vi "Run Bfr Tx - Check Valid Buffer.vi"(8 "error in (no error)":errorcluster, 11 "Tx Loop Data in":T1={"General Resources"={"Packet Name"="", "Packet ID"=0, "Local IP Address"="", "Local Port"=0, "Multicast"=FALSE, "Multicast IP Address"=0, "Header Info"=[], "Byte Order"=enum."big-endian, network order", "Channel Data Types"=[], "Duplex Packets"=refnum}, "Header Details"={"Packet Size"=0, "Protocol Revision"=0, "System Definition Version"=0, "Source Node Name"="", "Packet ID"=0, "Number of Channels"=0, "Static Header Size"=0, "Total Header Size"=0}, "Buffer Resources"={"Data Buffer"=0, "Pointer Encoding"=enum."Direct Encoding", "Buffer Size"=0, "Raw Buffer Data"=[], "Is Buffered"=FALSE, "External Buffer"=FALSE, "Prepend Header"=FALSE, "Valid Buffer"=FALSE}, "Runtime Resources"={"Connection ID"=refnum, "Transmit Option"=enum."Always", "Destination IP Address"=0, "Destination Port"=0, "Multicast IP Address"=0, "TTL"=0, "Multicast"=FALSE, "Port as Channel"=FALSE, "ExecutionConfig"={"Loop Period"=0, "RT Loop Period"=-2, "Untimed Period"=0, "Target Processor"=0, "Priority"=0, "Thread Management"=enum."Untimed (Default)"}}, "Echo Resources"={"Transmit Echo Option"=enum."PCL Reset", "Packet Count"=0.0, "Counter Increment"=0.0, "Transmit Values"=[]}, "Buffer Option Support"={"Buffer Option"=enum."Static Buffer", "Sim Option"=enum."No Simulation"}, "Channel Resources"={"Transmit Flag"=refnum, "Transmit Echo"=refnum, "Transmit Bytes"=refnum, "Port Channel"=refnum, "Buffer (External)"=refnum, "Buffer (Local)"=refnum, "Timestamp"=refnum}, "Debug Resources"={"Debug Mode"=FALSE, "Debug Log File"=refnum, "Packet Name"=""}} {"Buffer Resources"."Data Buffer" format="%016x"}) -> (0 "error out":errorcluster, 3 "Tx Loop Data out":T1={"General Resources"={"Packet Name"="", "Packet ID"=0, "Local IP Address"="", "Local Port"=0, "Multicast"=FALSE, "Multicast IP Address"=0, "Header Info"=[], "Byte Order"=enum."big-endian, network order", "Channel Data Types"=[], "Duplex Packets"=refnum}, "Header Details"={"Packet Size"=0, "Protocol Revision"=0, "System Definition Version"=0, "Source Node Name"="", "Packet ID"=0, "Number of Channels"=0, "Static Header Size"=0, "Total Header Size"=0}, "Buffer Resources"={"Data Buffer"=0, "Pointer Encoding"=enum."Direct Encoding", "Buffer Size"=0, "Raw Buffer Data"=[], "Is Buffered"=FALSE, "External Buffer"=FALSE, "Prepend Header"=FALSE, "Valid Buffer"=FALSE}, "Runtime Resources"={"Connection ID"=refnum, "Transmit Option"=enum."Always", "Destination IP Address"=0, "Destination Port"=0, "Multicast IP Address"=0, "TTL"=0, "Multicast"=FALSE, "Port as Channel"=FALSE, "ExecutionConfig"={"Loop Period"=0, "RT Loop Period"=-2, "Untimed Period"=0, "Target Processor"=0, "Priority"=0, "Thread Management"=enum."Untimed (Default)"}}, "Echo Resources"={"Transmit Echo Option"=enum."PCL Reset", "Packet Count"=0.0, "Counter Increment"=0.0, "Transmit Values"=[]}, "Buffer Option Support"={"Buffer Option"=enum."Static Buffer", "Sim Option"=enum."No Simulation"}, "Channel Resources"={"Transmit Flag"=refnum, "Transmit Echo"=refnum, "Transmit Bytes"=refnum, "Port Channel"=refnum, "Buffer (External)"=refnum, "Buffer (Local)"=refnum, "Timestamp"=refnum}, "Debug Resources"={"Debug Mode"=FALSE, "Debug Log File"=refnum, "Packet Name"=""}} {"Buffer Resources"."Data Buffer" format="%016x"})   [LabVIEW 2016, in "UDP-Custom-Device Engine.lvlib"]
uses:
  UDP-Custom-Device Engine.lvlib
  Types/Engine - Buffered Tx Loop Data.ctl
  Types/Engine - General Resources.ctl
  <vilib>/NI Veristand/VeriStand Data/Typedefs/Typedefs.Data Types.ctl
  Shared/Types/Shared - Duplex Settings.ctl
  Shared/Types/Shared - Header Details.ctl
  Types/Engine - Buffer Resources.ctl
  Shared/Types/Shared - Pointer Encoding.ctl
  Types/Engine - Tx Runtime Resources.ctl
  Shared/Types/Shared - Transmit Flag Options.ctl
  Types/Engine - Execution Config.ctl
  Shared/Types/Shared - Thread Management.ctl
  Types/Engine - Tx Echo Resources.ctl
  Shared/Types/Shared - Transmit Echo Options.ctl
  Types/Engine - Buffered Tx Buffer Option Support.ctl
  Shared/Types/Shared - Transmit Buffer Options.ctl
  Shared/Types/Shared - Transmit Sim Options.ctl
  Types/Engine - Buffered Tx Channel Refs.ctl
  <vilib>/NI/NIVS Inline Async API/_Data Access Engine/Data Access Engine/Types/Read.DVR.ctl
  <vilib>/NI/NIVS Inline Async API/_Data Access Engine/Access Type Classes/Read/Read.lvclass
  <vilib>/NI/NIVS Inline Async API/_Data Access Engine/Data Access Engine/Types/Write.DVR.ctl
  <vilib>/NI/NIVS Inline Async API/_Data Access Engine/Access Type Classes/Write/Write.lvclass
  Types/Engine - Debug Resources.ctl
  <vilib>/NI/NIVS Inline Async API/_Data Access Engine/Access Type Classes/Read/Read.lvclass/Read.ctl
  <vilib>/NI/NIVS Inline Async API/_Data Access Engine/Data Access Engine/Methods/Read.Data.vi
  <vilib>/NI/NIVS Inline Async API/_Data Access Engine/Access Type Classes/Read/Read.ProcessData.vi
  <vilib>/NI/NIVS Inline Async API/_Data Access Engine/Data Access Engine/Data Access Engine.lvclass
  Shared/UDP-Custom-Device Shared.lvlib
  <vilib>/NI Veristand/VeriStand Data/VeriStand Data.lvlib
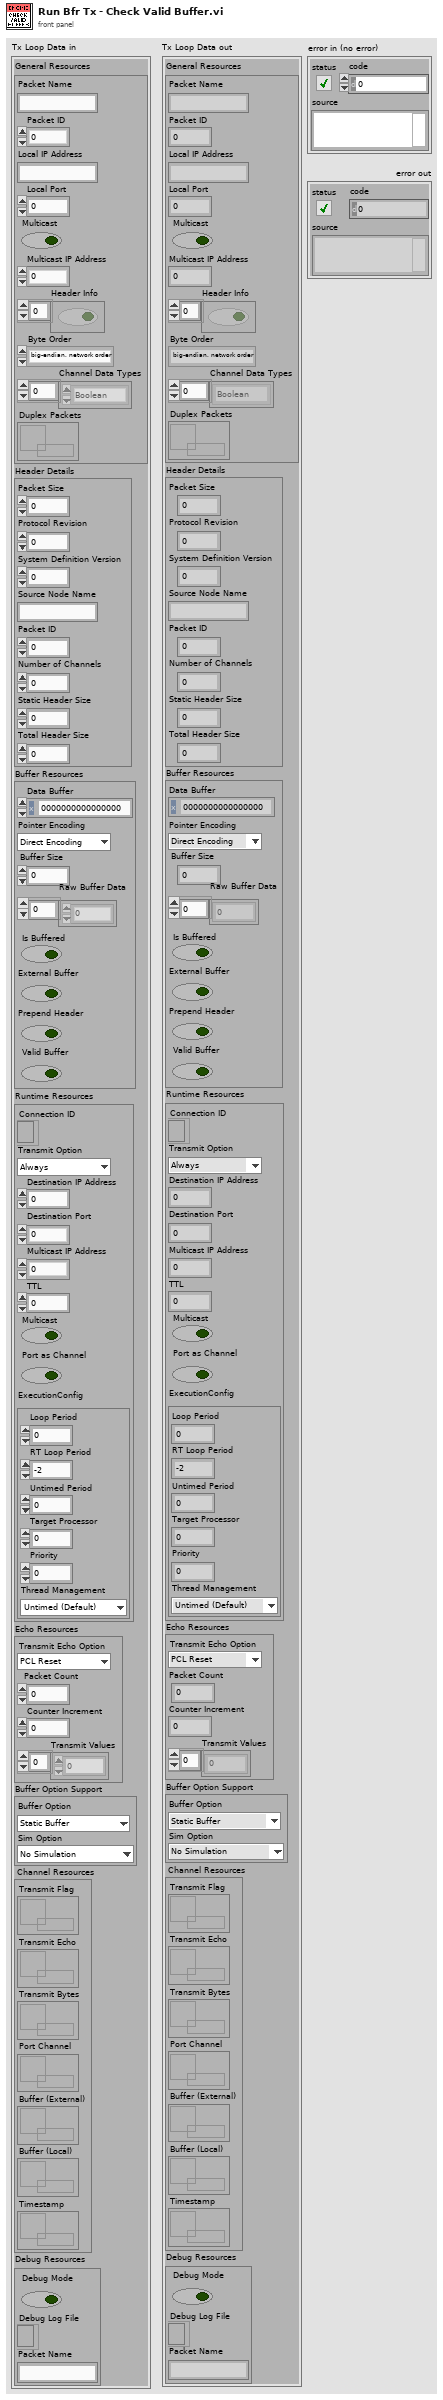
[diagram p1: front panel]
types:
  T1 = typedef "UDP-Custom-Device Engine.lvlib/Engine - Buffered Tx Loop Data.ctl" = cluster{"General Resources":T2, "Header Details":T4, "Buffer Resources":T5, "Runtime Resources":T7, "Echo Resources":T11, "Buffer Option Support":T13, "Channel Resources":T16, "Debug Resources":T19}
  T2 = typedef "UDP-Custom-Device Engine.lvlib/Engine - General Resources.ctl" = cluster{"Packet Name":string, "Packet ID":i32, "Local IP Address":string, "Local Port":i32, "Multicast":bool, "Multicast IP Address":u32, "Header Info":bool[], "Byte Order":enum16{"big-endian, network order", "native, host order", "little-endian"}, "Channel Data Types":T3[], "Duplex Packets":refnum<data-value>}
  T3 = typedef "VeriStand Data.lvlib/Typedefs.Data Types.ctl" = enum16{"Boolean", "Single", "Double", "I8", "I16", "I32", "I64", "U8", "U16", "U32", "U64"}
  T4 = typedef "UDP-Custom-Device Shared.lvlib/Shared - Header Details.ctl" = cluster{"Packet Size":u16, "Protocol Revision":u8, "System Definition Version":u64, "Source Node Name":string, "Packet ID":u32, "Number of Channels":u32, "Static Header Size":u16, "Total Header Size":u16}
  T5 = typedef "UDP-Custom-Device Engine.lvlib/Engine - Buffer Resources.ctl" = cluster{"Data Buffer":u64, "Pointer Encoding":T6, "Buffer Size":u64, "Raw Buffer Data":u8[], "Is Buffered":bool, "External Buffer":bool, "Prepend Header":bool, "Valid Buffer":bool}
  T6 = typedef "UDP-Custom-Device Shared.lvlib/Shared - Pointer Encoding.ctl" = enum16{"Direct Encoding", "Conversion Encoding"}
  T7 = typedef "UDP-Custom-Device Engine.lvlib/Engine - Tx Runtime Resources.ctl" = cluster{"Connection ID":refnum<k16>, "Transmit Option":T8, "Destination IP Address":u32, "Destination Port":u16, "Multicast IP Address":u32, "TTL":u16, "Multicast":bool, "Port as Channel":bool, "ExecutionConfig":T9}
  T8 = typedef "UDP-Custom-Device Shared.lvlib/Shared - Transmit Flag Options.ctl" = enum16{"Always", "One-Shot", "Toggle"}
  T9 = typedef "UDP-Custom-Device Engine.lvlib/Engine - Execution Config.ctl" = cluster{"Loop Period":i64, "RT Loop Period":i64, "Untimed Period":u32, "Target Processor":i32, "Priority":i32, "Thread Management":T10}
  T10 = typedef "UDP-Custom-Device Shared.lvlib/Shared - Thread Management.ctl" = enum16{"Untimed (Default)", "Timed (High Priority)"}
  T11 = typedef "UDP-Custom-Device Engine.lvlib/Engine - Tx Echo Resources.ctl" = cluster{"Transmit Echo Option":T12, "Packet Count":dbl, "Counter Increment":dbl, "Transmit Values":dbl[]}
  T12 = typedef "UDP-Custom-Device Shared.lvlib/Shared - Transmit Echo Options.ctl" = enum16{"PCL Reset", "Counter", "Mirror"}
  T13 = typedef "UDP-Custom-Device Engine.lvlib/Engine - Buffered Tx Buffer Option Support.ctl" = cluster{"Buffer Option":T14, "Sim Option":T15}
  T14 = typedef "UDP-Custom-Device Shared.lvlib/Shared - Transmit Buffer Options.ctl" = enum16{"Static Buffer", "FIFO Buffer", "FIFO Buffer + Port"}
  T15 = typedef "UDP-Custom-Device Shared.lvlib/Shared - Transmit Sim Options.ctl" = enum16{"No Simulation", "Counter", "Full Buffer", "FIFO Test", "FIFO + Port Test"}
  T16 = typedef "UDP-Custom-Device Engine.lvlib/Engine - Buffered Tx Channel Refs.ctl" = cluster{"Transmit Flag":T17, "Transmit Echo":T18, "Transmit Bytes":T17, "Port Channel":T17, "Buffer (External)":T17, "Buffer (Local)":T18, "Timestamp":T17}
  T17 = typedef "Data Access Engine.lvlib/Data Access Engine.lvclass/Read.DVR.ctl" = refnum<data-value>
  T18 = typedef "Data Access Engine.lvlib/Data Access Engine.lvclass/Write.DVR.ctl" = refnum<data-value>
  T19 = typedef "UDP-Custom-Device Engine.lvlib/Engine - Debug Resources.ctl" = cluster{"Debug Mode":bool, "Debug Log File":refnum<file>, "Packet Name":string}
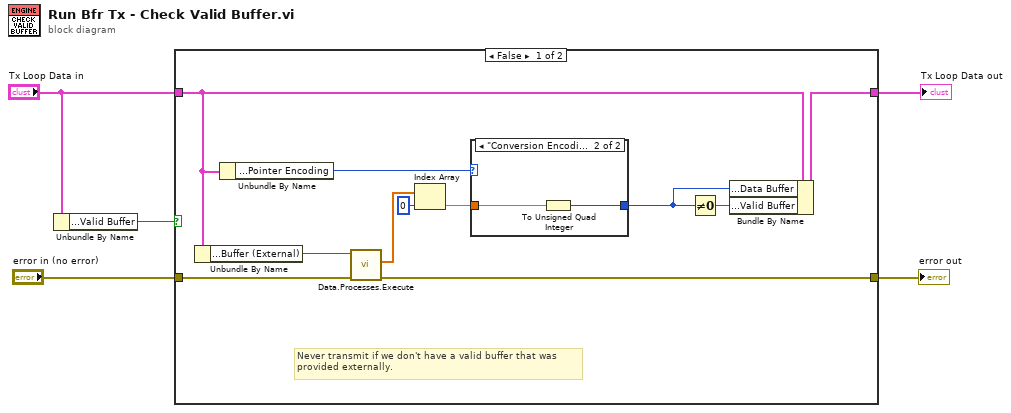
[diagram p0: block diagram]
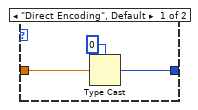
[diagram p2: hidden frame]
diagram:
  n1 = Unbundle By Name("Tx Loop Data in") -> ("Buffer Resources.Valid Buffer"=w2:bool)
  n2 = case shown="False" w2 {
    tunnel: "Tx Loop Data in" -> [w7 w23]
    tunnel: "error in (no error)" -> [w15 w22]
    tunnel: [w14 w22] -> w4
    tunnel: [w11 w23] -> w1
    frame False {
      # "Never transmit if we don't have a valid buffer that was\nprovided externally."
      n3 = Unbundle By Name(w7) -> ("Channel Resources.Buffer (External)"=w16:T17)
      n4 = Unbundle By Name(w7) -> ("Buffer Resources.Pointer Encoding"=w6:T6)
      n5 = call-poly <vilib>:"Data.Processes.Execute.vi"("error in (no error)"=w15, "Ref"=w16) -> ("error out"=w14:errorcluster, "Values"=w13:dbl[])  [unwired: 7 in, 1 out]
      n6 = Index Array(array=w13, index=0) -> (element=w9:dbl)
      n7 = case shown="\"Conversion Encoding\"" w6 {
        tunnel: w9 -> [w19 w21]
        tunnel: [w18 w20] -> w8
        frame "Direct Encoding", Default {
          n8 = Type Cast(type=u64 0, x=w19) -> (*(type *) &x=w18:u64)
        }
        frame "Conversion Encoding" {
          n9 = To Unsigned Quad Integer(1:w21) -> (0:w20:u64)
        }
      }
      n10 = Not Equal To 0?(x=w8) -> (x != 0?=w10:bool)
      n11 = Bundle By Name(cluster=w7, "Buffer Resources.Data Buffer"=w8, "Buffer Resources.Valid Buffer"=w10) -> (w11:T1)
    }
    frame True {
      # "Does nothing once we have a valid buffer."
    }
  }
  "Tx Loop Data out" <- w1
  "error out" <- w4
